vi "ceciLV_loops.vi"() -> ()   [LabVIEW 2017]
panel:
  out "i (iteracion while) 3":i64
  out "i (iteracion while) 2":i64
  out "Sucesion 3":i64
  in  "Detener sucesion 2":bool
  out "Sucesion 2":i64
  out "i (iteracion for)":i64
  out "Sucesion":i64
  # "N VECES"
  # "CONDICION DE PARO"
  # "WHILE LOOP"
  # "FOR LOOP"
  # "2,4,6,8...(10 terminos)"
  # "Sucesion 2:\nEl usuario controla \ncuando se detiene\nel ciclo."
  # "Sucesion 3:\nSimilar al for, se detiene\ncuando llegue al 10mo\ntermino."
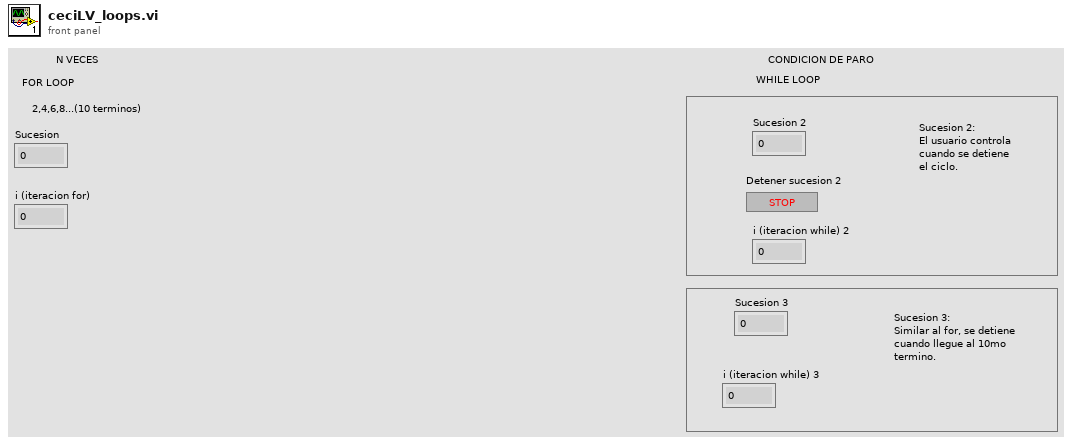
[diagram p1: front panel]
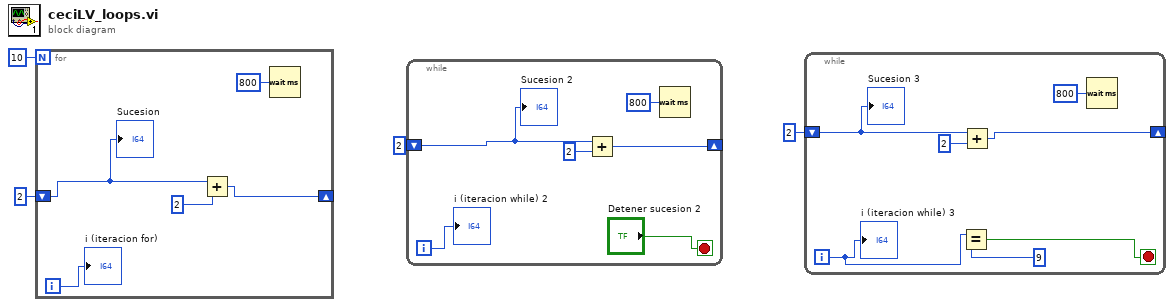
[diagram p0: block diagram]
diagram:
  n1 = for {
    N: 10 -> [_]
    shift-right: [w9] -> _
    shift-left: i64 2 -> [w7]
    i -> [w6]
    n2 = Add(x=w7, y=i64 2) -> (x+y=w9:i64)
    n3 = Wait (ms)(milliseconds to wait=u32 800) -> ()  [unwired: 1 out]
    "Sucesion" <- w7
    "i (iteracion for)" <- w6
  }
  n4 = while {
    shift-right: [w15] -> _
    shift-left: i64 2 -> [w13]
    i -> [w12]
    stop <- "Detener sucesion 2" stop-if-true
    n5 = Add(x=w13, y=i64 2) -> (x+y=w15:i64)
    n6 = Wait (ms)(milliseconds to wait=u32 800) -> ()  [unwired: 1 out]
    "Sucesion 2" <- w13
    "i (iteracion while) 2" <- w12
  }
  n7 = while {
    shift-right: [w22] -> _
    shift-left: i64 2 -> [w20]
    i -> [w19]
    stop <- w17 stop-if-true
    n8 = Equal?(x=w19, y=9) -> (x = y?=w17:bool)
    n9 = Add(x=w20, y=i64 2) -> (x+y=w22:i64)
    n10 = Wait (ms)(milliseconds to wait=u32 800) -> ()  [unwired: 1 out]
    "Sucesion 3" <- w20
    "i (iteracion while) 3" <- w19
  }
